vi "Read cal data.vi"(8 "error in (no error)":errorcluster, 11 "device_type in":refnum<class "device_type.lvclass">) -> (0 "error out":errorcluster, 1 "apply cal data":bool, 2 "cal data":T1(array[cluster]), 3 "device_type out":refnum<class "device_type.lvclass">)   [LabVIEW 2021, in "device_type.lvclass"]
uses:
  device_type.lvclass
  device_type.lvclass/device_type.ctl
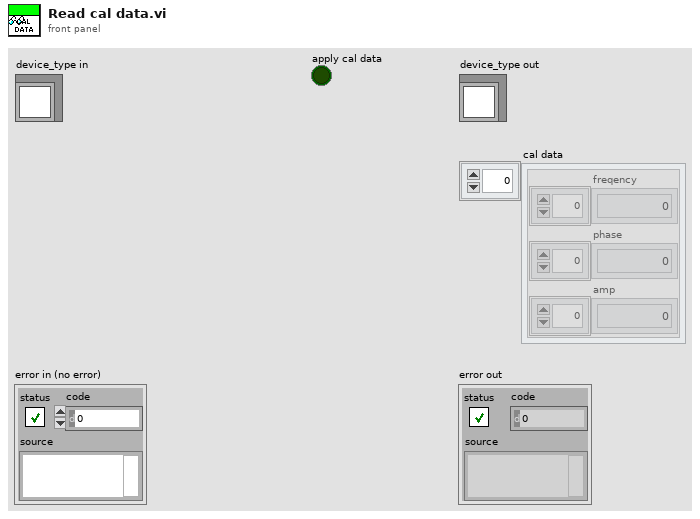
[diagram p1: front panel]
types:
  T1 = cluster{"freqency":dbl[], "phase":dbl[], "amp":dbl[]}[]
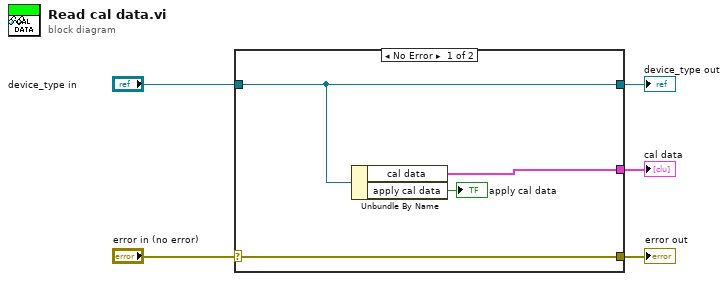
[diagram p0: block diagram]
diagram:
  n1 = case shown="No Error" "error in (no error)" {
    selector: "error in (no error)" -> [w9 w10]
    tunnel: [w9 w10] -> w4
    tunnel: [w8 w11] -> w2
    tunnel: "device_type in" -> [w8 w11]
    tunnel: [w7 _] -> w1
    frame No Error {
      n2 = Unbundle By Name(w8) -> ("cal data"=w7:T1, "apply cal data"=→"apply cal data":bool)
    }
    frame Error {
    }
  }
  "error out" <- w4
  "device_type out" <- w2
  "cal data" <- w1
